vi "Stop TCS Qeue.vi"(8 "error in (no error)":errorcluster, 11 "Channel in":refnum<class "Channel.lvclass">) -> (0 "error out":errorcluster, 3 "Channel out":refnum<class "Channel.lvclass">)   [LabVIEW 2018, in "Channel.lvclass"]
uses:
  Channel.lvclass
  Channel.lvclass/Channel.ctl
  TCS/TCS.lvclass
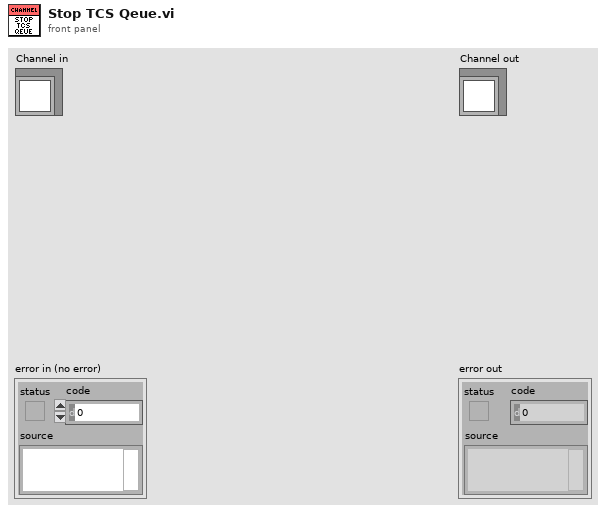
[diagram p1: front panel]
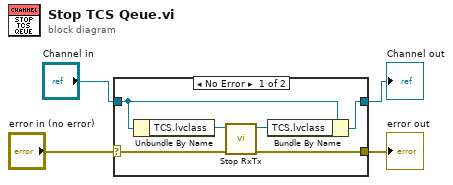
[diagram p0: block diagram]
diagram:
  n1 = case shown="No Error" "error in (no error)" {
    selector: "error in (no error)" -> [w6 w12]
    tunnel: [w5 w12] -> w3
    tunnel: [w8 w11] -> w1
    tunnel: "Channel in" -> [w9 w11]
    frame No Error {
      n2 = Unbundle By Name(w9) -> ("TCS.lvclass"=w10:refnum<class "TCS.lvclass">)
      n3 = call "Stop RxTx.vi"("error in (no error)"=w6, "TCS in"=w10) -> ("error out"=w5:errorcluster, "TCS out"=w7:refnum<class "TCS.lvclass">)  [unwired: 8 in]
      n4 = Bundle By Name(cluster=w9, "TCS.lvclass"=w7) -> (w8:refnum<class "Channel.lvclass">)
    }
    frame Error {
    }
  }
  "error out" <- w3
  "Channel out" <- w1
